vi "FindRequiringComponents.vi"(4 "Item Types (all visible)":T4 items=["all visible", "all including hidden", "standard only", "startup only"], 5 "Component Version":string, 6 "Version Selection Modes":u32[](array[numeric]), 7 "Software IDs to Uninstall":string[](array[string]), 8 "error in (no error)":errorcluster, 9 "Software to Install":T3[](array[typedef]) {"component type" items=["standard", "hidden", "system", "unknown", "startup", "image"]}, 10 "Component ID":string, 11 "Session in":refnum<k21>) -> (0 "error out":errorcluster, 2 "Requiring Components":T1[](array[typedef]) {"Visibility Type" items=["standard", "hidden", "system", "unknown", "startup", "image"]}, 3 "Session out":refnum<k21>)   [LabVIEW 2014, in "nisyscfg.lvlib"]
uses:
  nisyscfg.lvlib
  Component Types.ctl
  Software 1.2.ctl
  Component Type.ctl
  Software Extended.ctl
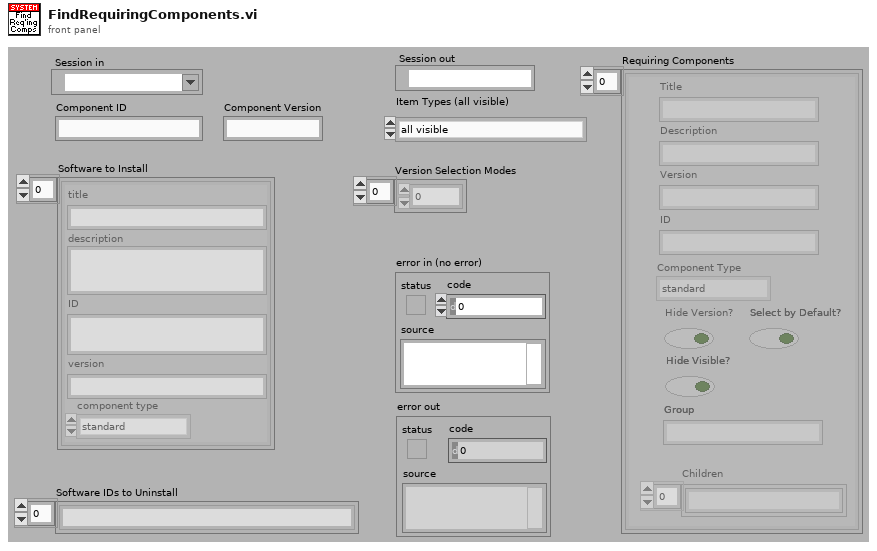
[diagram p1: front panel]
types:
  T1 = typedef "nisyscfg.lvlib/Software Extended.ctl" = cluster{"Description":string, "ID":string, "Version":string, "Title":string, "Visibility Type":T2, "Hide Version?":bool, "Children":string[], "Select by Default?":bool, "Hide Visible?":bool, "Group":string}
  T2 = typedef "nisyscfg.lvlib/Component Type.ctl" = u32
  T3 = typedef "nisyscfg.lvlib/Software 1.2.ctl" = cluster{"title":string, "description":string, "ID":string, "version":string, "component type":T2}
  T4 = typedef "nisyscfg.lvlib/Component Types.ctl" = u32
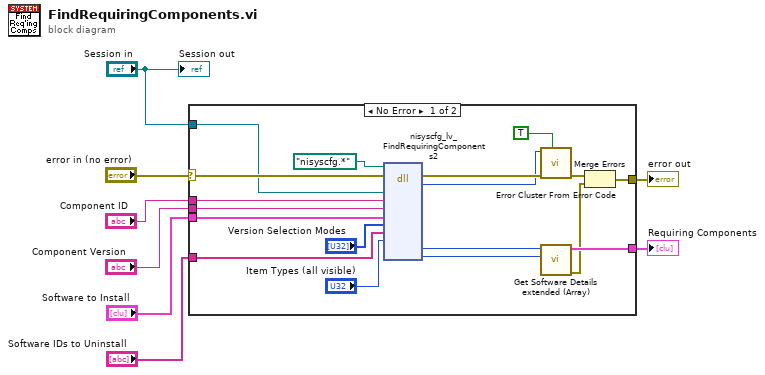
[diagram p0: block diagram]
diagram:
  n1 = case shown="No Error" "error in (no error)" {
    selector: "error in (no error)" -> [w24 w27]
    tunnel: "Session in" -> [w23 _]
    tunnel: "Component Version" -> [w21 _]
    tunnel: "Component ID" -> [w20 _]
    tunnel: [w14 w27] -> w4
    tunnel: "Software to Install" -> [w18 _]
    tunnel: "Software IDs to Uninstall" -> [w17 _]
    tunnel: [w12 _] -> w1
    frame No Error {
      n2 = dll-call lib="nisyscfg.*" fn="nisyscfg_lv_FindRequiringComponents2" label="FindRequiringComponents"(path in=path "nisyscfg.*", error in=w24, "session"=w23, "componentID"=w20, "componentVersion"=w21, "softwareToInstall"=w18, "versionSelectionMode"="Version Selection Modes", "softwareIDsToUninstall"=w17, "includeTypes"="Item Types (all visible)") -> (error out=w26:errorcluster, "result"=w25:i32, "requiringComponents"=w13:u64, "numComponents"=w10:i32)  [unwired: 10 in, 1 out]
      n3 = call "Error Cluster From Error Code.vi"("show call chain? (False)"=TRUE, "error in (no error)"=w26, "error code (0)"=w25) -> ("error out"=w15:errorcluster)  [unwired: 6 in]
      n4 = call "Get Software Details extended (Array).vi"("Number of Elements"=w10, "Enumerator in"=w13) -> ("error out"=w11:errorcluster, "Software Components"=w12:T1[])  [unwired: 8 in]
      n5 = Merge Errors(w15, w11) -> (w14:errorcluster)
    }
    frame Error {
    }
  }
  "error out" <- w4
  "Requiring Components" <- w1
  "Session out" <- "Session in"
